vi "Read Trigger.vi"(8 "error in (no error)":errorcluster, 11 "CCDCamera in":refnum<class "Simulated_CCD_Camera.lvclass">) -> (0 "error out":errorcluster, 2 "Trigger":u16(ring) items=["Internal", "External", "-", "-", "-", "-", "External Start"], 3 "CCDCamera out":refnum<class "Simulated_CCD_Camera.lvclass">)   [LabVIEW 2018, in "Simulated_CCD_Camera.lvclass"]
uses:
  Simulated_CCD_Camera.lvclass
  Simulated_CCD_Camera.lvclass/Simulated_CCD_Camera.ctl
  Interface/Interface.lvclass
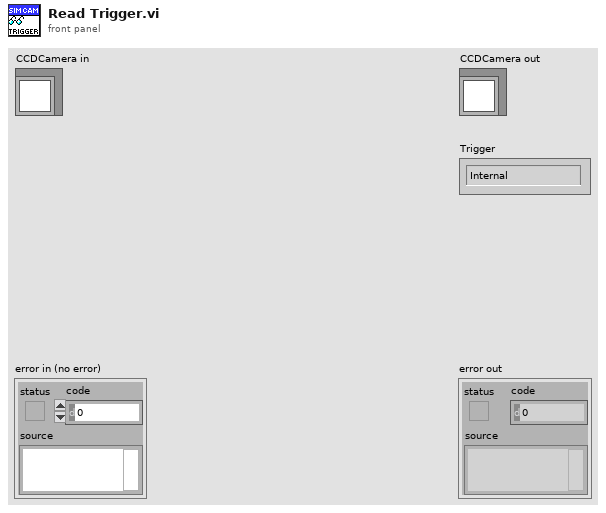
[diagram p1: front panel]
types:
  T1 = typedef "Shutter_mode typedef.ctl" = enum16{"Auto", "Open", "Close", "N/A (3)", "Open FVB Series", "Open Any Series"}
  T2 = typedef "ReadMode_mode typedef.ctl" = enum16{"Full Vertical Binning", "Multi-Track", "Random-Track", "Single-Track", "Image"}
  T3 = typedef "AcquisitionMode_mode typedef.ctl" = enum16{"Reserved (0)", "Single Scan", "Accumulate", "Kinetics", "Fast Kinetics", "Run Till Abort", "Reserved (6)", "Reserved (7)", "Reserved (8)", "Time Delayed Integration"}
  T4 = cluster{"EXPTIME":sgl, "PREAMP":enum16{"Gain 1", "Gain 2"}, "READOUT_RATE":enum16{"1 MHz", "10 MHz", "20 MHz", "30 MHz"}, "EM_GAIN":u16, "VBIN":u16, "INITIAL_LINE":u16, "INITIAL_COLUMN":u16, "FINAL_LINE":u16, "FINAL_COLUMN":u16, "#FRAMES":u32, "#CUBES":u32, "TRIGGER_MODE":enum16{"Internal", "External", "N/A", "N/A_1", "N/A_2", "N/A_3", "External Start"}, "HBIN":u16, "SHUTTER_TTL":enum16{"TTL Low", "TTL High"}, "SHUTTER_MODE":T1, "SHUTTER_OPENING_TIME":u16, "SHUTTER_CLOSING_TIME":u16, "VERTICAL_SHIFT_SPEED":u16, "READ_MODE":T2, "FRAME_TRANSFER":bool, "VERTICAL_CLOCK_VOLTAGE":enum16{"0", "+1", "+2", "+3", "+4"}, "ACQUISITION_MODE":T3, "AD_CHANNEL":u16, "EM_MODE":enum16{"Electron Multiplying", "Conventional"}}
  T5 = enum16{"Internal", "External", "N/A", "N/A_1", "N/A_2", "N/A_3", "External Start"}
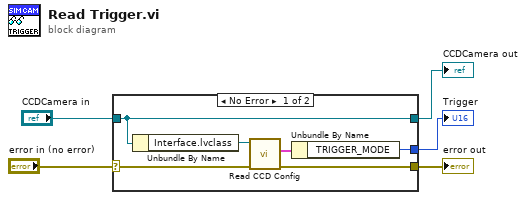
[diagram p0: block diagram]
diagram:
  n1 = case shown="No Error" "error in (no error)" {
    selector: "error in (no error)" -> [w7 w12]
    tunnel: [w6 w12] -> w4
    tunnel: [w11 w13] -> w2
    tunnel: "CCDCamera in" -> [w11 w13]
    tunnel: [w8 _] -> w1
    frame No Error {
      n2 = Unbundle By Name(w11) -> ("Interface.lvclass"=w10:refnum<class "Interface.lvclass">)
      n3 = call "Read CCD Config.vi"("error in (no error)"=w7, "Interface in"=w10) -> ("error out"=w6:errorcluster, "CCD Config"=w9:T4)  [unwired: 7 in, 1 out]
      n4 = Unbundle By Name(w9) -> ("TRIGGER_MODE"=w8:T5)
    }
    frame Error {
    }
  }
  "error out" <- w4
  "CCDCamera out" <- w2
  "Trigger" <- w1
